vi "UpdateWhy(SubVI).vi"(9 "QuestionsNo_Ordered":string, 11 "connection reference":T1) -> ()   [LabVIEW 2013]
uses:
  <vilib>/addons/database/Connection.llb/Conn ObjectReference.ctl
  FYP_LabviewGlobal(SubVI).vi
  <vilib>/addons/database/NI_Database_API.lvlib
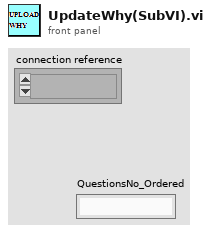
[diagram p1: front panel]
types:
  T1 = typedef "NI_Database_API.lvlib/Conn ObjectReference.ctl" = refnum<k1>
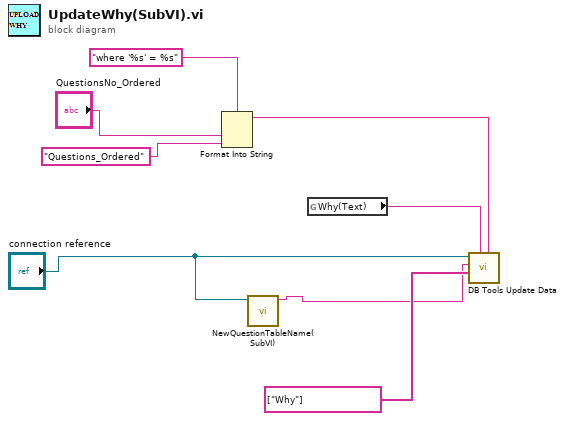
[diagram p0: block diagram]
diagram:
  n1 = Format Into String(format string="where '%s' = %s", "QuestionsNo_Ordered", "Questions_Ordered") -> (resulting string=w3:string)  [unwired: 2 in, 1 out]
  n2 = call "NewQuestionTableName(SubVI).vi"("connection reference"="connection reference") -> ("String"=w2:string)  [unwired: 9 in, 1 out]
  n3 = global read "FYP_LabviewGlobal(SubVI).vi" "Why(Text)"() -> (w7:string)
  n4 = call <vilib>:"DB Tools Update Data.vi"("condition"=w3, "data"=w7, "columns"=string[] ["Why"], "table"=w2, "connection reference"="connection reference") -> ()  [unwired: 5 in, 2 out]
